vi "Generic command handler.vi"(8 "error in (no error)":errorcluster, 10 "Message in":refnum<class "GenericMessage.lvclass">, 11 "StageSPIM in":refnum<class "StageSPIM.lvclass">) -> (0 "error out":errorcluster, 2 "value":string, 3 "StageSPIM out":refnum<class "StageSPIM.lvclass">)   [LabVIEW 2012, in "StageSPIM.lvclass"]
doc: "The generic_command_handler processes the command 'generic'. Commands which are not part of the predefined list of commands fall under the 'generic' command for special activity."
uses:
  StageSPIM.lvclass
  <vilib>/Distrio/Murmex/GenericMessage/GenericMessage.lvclass
  <vilib>/Distrio/Murmex/Murmex/Murmex.lvclass
  StageSPIM.lvclass/StageSPIM.ctl
  <vilib>/Distrio/Murmex/ProceedMessage/ProceedMessage.lvclass
  <vilib>/Distrio/Murmex/Message/Message.lvclass
panel:
  # "This method is called when the GENERIC\ntrigger is sent. \n\nOverride this method when your component needs to\nrespond to this trigger. \n\nCall parent for proper implementation"
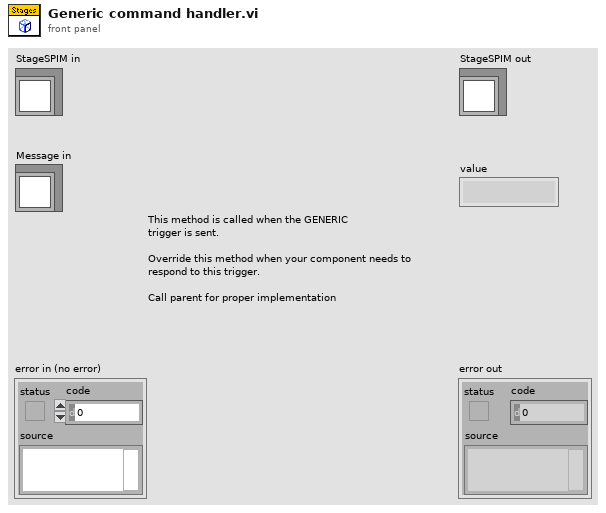
[diagram p1: front panel]
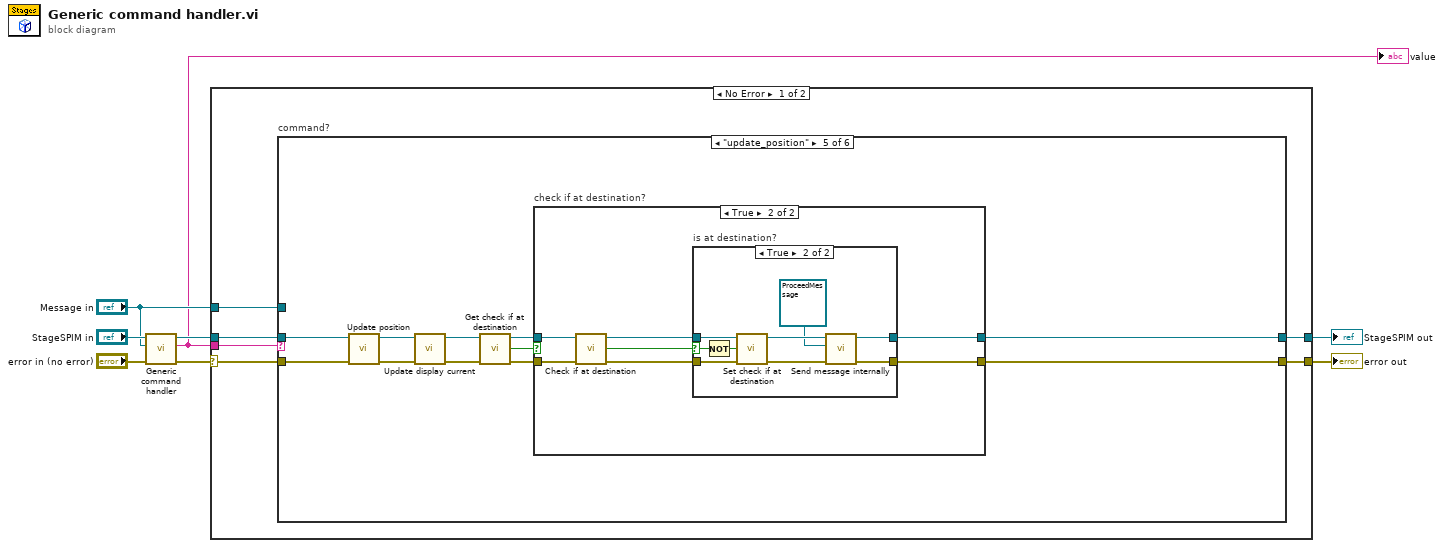
[diagram p0: block diagram]
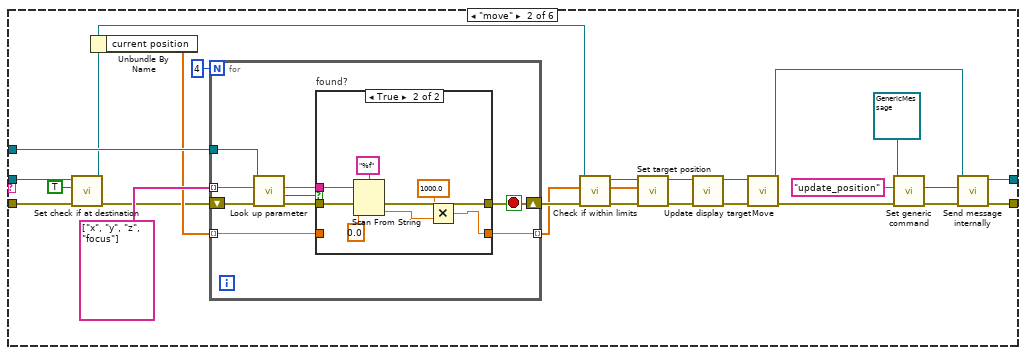
[diagram p3: hidden frame]
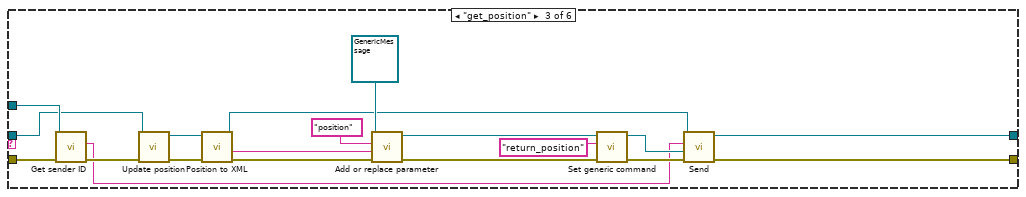
[diagram p5: hidden frame]
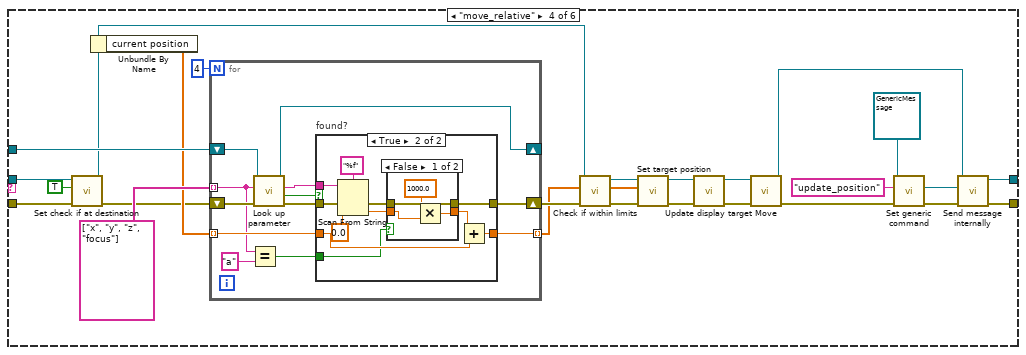
[diagram p6: hidden frame]
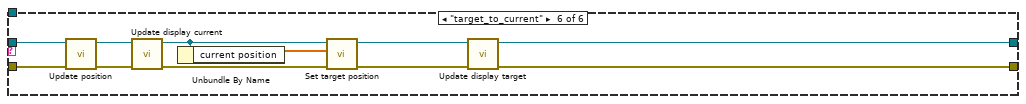
[diagram p11: hidden frame]
diagram:
  n1 = call-parent "Generic command handler.vi"("error in (no error)"="error in (no error)", "Message in"="Message in", "Murmex in"="StageSPIM in") -> ("error out"=w6:errorcluster, "value"=w3:string, "Murmex out"=w5:refnum<class "StageSPIM.lvclass">)  [unwired: 6 in]
  "value" <- w3
  n2 = case shown="No Error" w6 {
    selector: w6 -> [w13 w180]
    tunnel: w3 -> [w14 _]
    tunnel: w5 -> [w12 w181]
    tunnel: "Message in" -> [w11 _]
    tunnel: [w10 w180] -> w2
    tunnel: [w9 w181] -> w1
    frame No Error {
      n3 = case "command?" shown="\"update_position\"" w14 {
        tunnel: w13 -> [w15 w31 w80 w95 w148 w177]
        tunnel: w12 -> [w16 w33 w66 w97 w147 w176]
        tunnel: w11 -> [_ w38 w79 w102 _ _]
        tunnel: [w15 w24 w62 w88 w142 w171] -> w10
        tunnel: [w16 w21 w63 w85 w143 w169] -> w9
        frame Default {
        }
        frame "move" {
          n4 = call-dynamic "Set check if at destination.vi"("error in (no error)"=w31, "check if at destination"=TRUE, "StageSPIM in"=w33) -> ("error out"=w30:errorcluster, "StageSPIM out"=w32:refnum<class "StageSPIM.lvclass">)  [unwired: 7 in]
          n5 = Unbundle By Name(w32) -> ("current position"=w35:dbl[])
          n6 = for {
            N: 4 -> [_]
            shift-right: [w44] -> w39
            shift-left: w30 -> [w51]
            tunnel: string[] ["x", "y", "z", "focus"] -> [w43] mode=indexing
            tunnel: w35 -> [w46] mode=indexing
            tunnel: [w45] -> w34 mode=indexing
            tunnel: w38 -> [w47]
            stop <- w44 stop-if-true
            n7 = call <vilib>:"Look up parameter.vi"("error in (no error)"=w51, "name"=w43, "Message in"=w47) -> ("error out"=w50:errorcluster, "found?"=w49:bool, "key"=w48:string)  [unwired: 5 in, 1 out]
            n8 = case "found?" shown="True" w49 {
              tunnel: w50 -> [w53 w61]
              tunnel: [w53 w57] -> w44
              tunnel: w48 -> [_ w59]
              tunnel: [w52 w55] -> w45
              tunnel: w46 -> [w52 _]
              frame False {
              }
              frame True {
                n9 = Scan From String(format string="%f", input string=w59, error in=w61, default 1=0.0 ("default value 1")) -> (error out=w57:errorcluster, output 1=w56:dbl)  [unwired: 1 in, 2 out]
                n10 = Multiply(x=1000.0, y=w56) -> (x*y=w55:dbl)
              }
            }
          }
          n11 = call-dynamic "Check if within limits.vi"("error in (no error)"=w39, "Position array in"=w34, "StageSPIM in"=w32) -> ("error out"=w41:errorcluster, "Approved postion array"=w40:dbl[], "StageSPIM out"=w42:refnum<class "StageSPIM.lvclass">)  [unwired: 4 in, 2 out]
          n12 = call-dynamic "Set target position.vi"("error in (no error)"=w41, "target position"=w40, "StageSPIM in"=w42) -> ("error out"=w20:errorcluster, "StageSPIM out"=w18:refnum<class "StageSPIM.lvclass">)  [unwired: 7 in]
          n13 = call-dynamic "Update display target.vi"("error in (no error)"=w20, "StageSPIM in"=w18) -> ("error out"=w19:errorcluster, "StageSPIM out"=w17:refnum<class "StageSPIM.lvclass">)  [unwired: 8 in]
          n14 = call-dynamic "Move.vi"("error in (no error)"=w19, "StageSPIM in"=w17) -> ("error out"=w28:errorcluster, "StageSPIM out"=w22:refnum<class "StageSPIM.lvclass">)  [unwired: 8 in]
          n15 = call <vilib>:"Set generic command.vi"("error in (no error)"=w28, "generic command"="update_position", "GenericMessage in"=refnum<class "GenericMessage.lvclass"> refnum ("Distrio Murmex 1.1:GenericMessage")) -> ("error out"=w27:errorcluster, "GenericMessage out"=w23:refnum<class "GenericMessage.lvclass">)  [unwired: 7 in]
          n16 = call <vilib>:"Send message internally.vi"("error in (no error)"=w27, "Message"=w23, "Murmex in"=w22) -> ("error out"=w24:errorcluster, "Murmex out"=w21:refnum<class "StageSPIM.lvclass">)  [unwired: 7 in]
        }
        frame "get_position" {
          n17 = call <vilib>:"Get sender ID.vi"("error in (no error)"=w80, "Message in"=w79) -> ("error out"=w78:errorcluster, "sender"=w74:string)  [unwired: 7 in, 1 out]
          n18 = call-dynamic "Update position.vi"("error in (no error)"=w78, "StageSPIM in"=w66) -> ("error out"=w68:errorcluster, "StageSPIM out"=w65:refnum<class "StageSPIM.lvclass">)  [unwired: 8 in]
          n19 = call-dynamic "Position to XML.vi"("error in (no error)"=w68, "StageSPIM in"=w65) -> ("error out"=w67:errorcluster, "XML string"=w64:string, "StageSPIM out"=w69:refnum<class "StageSPIM.lvclass">)  [unwired: 7 in]
          n20 = call <vilib>:"Add or replace parameter.vi"("error in (no error)"=w67, "value"=w64, "name"="position", "Message in"=refnum<class "GenericMessage.lvclass"> refnum ("Distrio Murmex 1.1:GenericMessage")) -> ("error out"=w72:errorcluster, "Message out"=w71:refnum<class "GenericMessage.lvclass">)  [unwired: 6 in]
          n21 = call <vilib>:"Set generic command.vi"("error in (no error)"=w72, "generic command"="return_position", "GenericMessage in"=w71) -> ("error out"=w76:errorcluster, "GenericMessage out"=w75:refnum<class "GenericMessage.lvclass">)  [unwired: 7 in]
          n22 = call <vilib>:"Send.vi"("error in (no error)"=w76, "Message"=w75, "recipient"=w74, "Murmex in"=w69) -> ("error out"=w62:errorcluster, "Murmex out"=w63:refnum<class "StageSPIM.lvclass">)  [unwired: 6 in]
        }
        frame "move_relative" {
          n23 = call-dynamic "Set check if at destination.vi"("error in (no error)"=w95, "check if at destination"=TRUE, "StageSPIM in"=w97) -> ("error out"=w94:errorcluster, "StageSPIM out"=w96:refnum<class "StageSPIM.lvclass">)  [unwired: 7 in]
          n24 = Unbundle By Name(w96) -> ("current position"=w99:dbl[])
          n25 = for {
            N: 4 -> [_]
            shift-right: [w115] -> w103
            shift-left: w94 -> [w118]
            tunnel: string[] ["x", "y", "z", "focus"] -> [w109] mode=indexing
            shift-right: [w112] -> _
            shift-left: w102 -> [w113]
            tunnel: w99 -> [w111] mode=indexing
            tunnel: [w110] -> w98 mode=indexing
            n26 = Equal?(x=w109, y="a") -> (x = y?=w107:bool)
            n27 = call <vilib>:"Look up parameter.vi"("error in (no error)"=w118, "name"=w109, "Message in"=w113) -> ("error out"=w117:errorcluster, "found?"=w116:bool, "key"=w114:string, "Message out"=w112:refnum<class "GenericMessage.lvclass">)  [unwired: 5 in]
            n28 = case "found?" shown="True" w116 {
              tunnel: w117 -> [w120 w131]
              tunnel: [w120 w124] -> w115
              tunnel: w114 -> [_ w129]
              tunnel: [w119 w127] -> w110
              tunnel: w111 -> [w119 w126]
              tunnel: w107 -> [_ w125]
              frame False {
              }
              frame True {
                n29 = Scan From String(format string="%f", input string=w129, error in=w131, default 1=0.0 ("default value 1")) -> (error out=w123:errorcluster, output 1=w121:dbl)  [unwired: 1 in, 2 out]
                n30 = case shown="False" w125 {
                  tunnel: [w135 w137] -> w124
                  tunnel: w123 -> [w135 w137]
                  tunnel: [w134 w136] -> w122
                  tunnel: w121 -> [w133 w136]
                  frame False {
                    n31 = Multiply(x=1000.0, y=w133) -> (x*y=w134:dbl)
                  }
                  frame True {
                  }
                }
                n32 = Add(x=w122, y=w126) -> (x+y=w127:dbl)
              }
            }
          }
          n33 = call-dynamic "Check if within limits.vi"("error in (no error)"=w103, "Position array in"=w98, "StageSPIM in"=w96) -> ("error out"=w105:errorcluster, "Approved postion array"=w104:dbl[], "StageSPIM out"=w106:refnum<class "StageSPIM.lvclass">)  [unwired: 4 in, 2 out]
          n34 = call-dynamic "Set target position.vi"("error in (no error)"=w105, "target position"=w104, "StageSPIM in"=w106) -> ("error out"=w84:errorcluster, "StageSPIM out"=w81:refnum<class "StageSPIM.lvclass">)  [unwired: 7 in]
          n35 = call-dynamic "Update display target.vi"("error in (no error)"=w84, "StageSPIM in"=w81) -> ("error out"=w83:errorcluster, "StageSPIM out"=w82:refnum<class "StageSPIM.lvclass">)  [unwired: 8 in]
          n36 = call-dynamic "Move.vi"("error in (no error)"=w83, "StageSPIM in"=w82) -> ("error out"=w92:errorcluster, "StageSPIM out"=w86:refnum<class "StageSPIM.lvclass">)  [unwired: 8 in]
          n37 = call <vilib>:"Set generic command.vi"("error in (no error)"=w92, "generic command"="update_position", "GenericMessage in"=refnum<class "GenericMessage.lvclass"> refnum ("Distrio Murmex 1.1:GenericMessage")) -> ("error out"=w91:errorcluster, "GenericMessage out"=w87:refnum<class "GenericMessage.lvclass">)  [unwired: 7 in]
          n38 = call <vilib>:"Send message internally.vi"("error in (no error)"=w91, "Message"=w87, "Murmex in"=w86) -> ("error out"=w88:errorcluster, "Murmex out"=w85:refnum<class "StageSPIM.lvclass">)  [unwired: 7 in]
        }
        frame "update_position" {
          n39 = call-dynamic "Update position.vi"("error in (no error)"=w148, "StageSPIM in"=w147) -> ("error out"=w141:errorcluster, "StageSPIM out"=w139:refnum<class "StageSPIM.lvclass">)  [unwired: 8 in]
          n40 = call-dynamic "Update display current.vi"("error in (no error)"=w141, "StageSPIM in"=w139) -> ("error out"=w140:errorcluster, "StageSPIM out"=w138:refnum<class "StageSPIM.lvclass">)  [unwired: 8 in]
          n41 = call-dynamic "Get check if at destination.vi"("error in (no error)"=w140, "StageSPIM in"=w138) -> ("error out"=w145:errorcluster, "check if at destination"=w146:bool, "StageSPIM out"=w144:refnum<class "StageSPIM.lvclass">)  [unwired: 7 in]
          n42 = case "check if at destination?" shown="True" w146 {
            tunnel: w145 -> [w150 w157]
            tunnel: w144 -> [w149 w156]
            tunnel: [w149 w152] -> w143
            tunnel: [w150 w151] -> w142
            frame False {
            }
            frame True {
              n43 = call-dynamic "Check if at destination.vi"("error in (no error)"=w157, "StageSPIM in"=w156) -> ("error out"=w154:errorcluster, "at destination?"=w155:bool, "StageSPIM out"=w153:refnum<class "StageSPIM.lvclass">)  [unwired: 7 in]
              n44 = case "is at destination?" shown="True" w155 {
                selector: w155 -> [_ w167]
                tunnel: w154 -> [w159 w168]
                tunnel: w153 -> [w158 w165]
                tunnel: [w159 w161] -> w151
                tunnel: [w158 w160] -> w152
                frame False {
                }
                frame True {
                  n45 = Not(x=w167) -> (.not. x?=w166:bool)
                  n46 = call-dynamic "Set check if at destination.vi"("error in (no error)"=w168, "check if at destination"=w166, "StageSPIM in"=w165) -> ("error out"=w164:errorcluster, "StageSPIM out"=w163:refnum<class "StageSPIM.lvclass">)  [unwired: 7 in]
                  n47 = call <vilib>:"Send message internally.vi"("error in (no error)"=w164, "Message"=refnum<class "ProceedMessage.lvclass"> refnum ("Distrio Murmex 1.1:ProceedMessage"), "Murmex in"=w163) -> ("error out"=w161:errorcluster, "Murmex out"=w160:refnum<class "StageSPIM.lvclass">)  [unwired: 7 in]
                }
              }
            }
          }
        }
        frame "target_to_current" {
          n48 = call-dynamic "Update position.vi"("error in (no error)"=w177, "StageSPIM in"=w176) -> ("error out"=w179:errorcluster, "StageSPIM out"=w178:refnum<class "StageSPIM.lvclass">)  [unwired: 8 in]
          n49 = call-dynamic "Update display current.vi"("error in (no error)"=w179, "StageSPIM in"=w178) -> ("error out"=w174:errorcluster, "StageSPIM out"=w175:refnum<class "StageSPIM.lvclass">)  [unwired: 8 in]
          n50 = Unbundle By Name(w175) -> ("current position"=w173:dbl[])
          n51 = call-dynamic "Set target position.vi"("error in (no error)"=w174, "target position"=w173, "StageSPIM in"=w175) -> ("error out"=w172:errorcluster, "StageSPIM out"=w170:refnum<class "StageSPIM.lvclass">)  [unwired: 7 in]
          n52 = call-dynamic "Update display target.vi"("error in (no error)"=w172, "StageSPIM in"=w170) -> ("error out"=w171:errorcluster, "StageSPIM out"=w169:refnum<class "StageSPIM.lvclass">)  [unwired: 8 in]
        }
      }
    }
    frame Error {
    }
  }
  "error out" <- w2
  "StageSPIM out" <- w1
